vi "RegTestInfo.vi"(9 "Key Definitions":string[](array[string])=["Job Number", "Unit Number", "Serial Number", "Technician", "Notes", "Config Path", "Report Path"], 10 "Mode":enum16{"Write", "Read", "Delete"}(ring), 11 "Key Value In":T1) -> (3 "Key Value out":string[](array[string]))   [LabVIEW 2024]
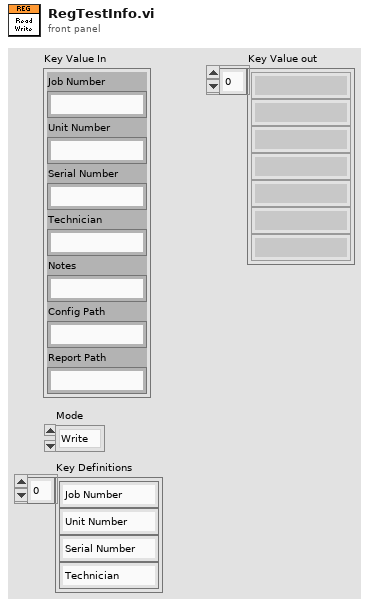
[diagram p1: front panel]
types:
  T1 = cluster{"Job Number":string, "Unit Number":string, "Serial Number":string, "Technician":string, "Notes":string, "Config Path":string, "Report Path":string}
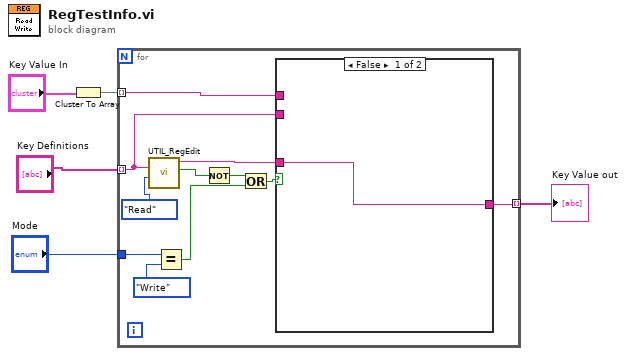
[diagram p0: block diagram]
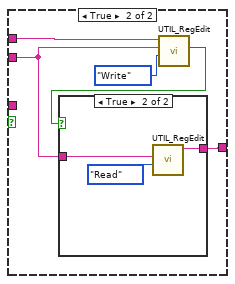
[diagram p2: hidden frame]
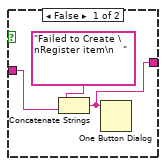
[diagram p3: hidden frame]
diagram:
  n1 = Cluster To Array(cluster="Key Value In") -> (array=w3:string[])
  n2 = for {
    tunnel: w3 -> [w15] mode=indexing
    tunnel: "Key Definitions" -> [w16] mode=indexing
    tunnel: [w14] -> w5 mode=indexing
    tunnel: "Mode" -> [w11]
    n3 = call "UTIL_RegEdit.vi"("Mode"=enum16{"Write", "Read", "Delete"}."Read", "String Name"=w16) -> ("Success?"=w7:bool, "Value Read"=w13:string)  [unwired: 8 in]
    n4 = Equal?(x=w11, y=enum16{"Write", "Read", "Delete"}."Write") -> (x = y?=w9:bool)
    n5 = Not(x=w7) -> (.not. x?=w6:bool)
    n6 = Or(x=w6, y=w9) -> (x .or. y?=w8:bool)
    n7 = case shown="False" w8 {
      tunnel: w16 -> [_ w20]
      tunnel: w15 -> [_ w21]
      tunnel: [w17 w19] -> w14
      tunnel: w13 -> [w17 _]
      frame False {
      }
      frame True {
        n8 = call "UTIL_RegEdit.vi"("Mode"=enum16{"Write", "Read", "Delete"}."Write", "String Name"=w20, "String Value"=w21) -> ("Success?"=w18:bool)  [unwired: 7 in, 1 out]
        n9 = case shown="True" w18 {
          tunnel: w20 -> [w24 w27]
          tunnel: [w23 w26] -> w19
          frame False {
            n10 = Concatenate Strings("Failed to Create \nRegister item\n   " ("message"), w24) -> (w23:string)
            n11 = One Button Dialog(message=w23) -> ()  [unwired: 1 in, 1 out]
          }
          frame True {
            n12 = call "UTIL_RegEdit.vi"("Mode"=enum16{"Write", "Read", "Delete"}."Read", "String Name"=w27) -> ("Value Read"=w26:string)  [unwired: 8 in, 1 out]
          }
        }
      }
    }
  }
  "Key Value out" <- w5
